vi "Stream Data.vi"(8 "error in (no error)":errorcluster, 10 "Data Type":string, 11 "Communication in":refnum<class "Communication.lvclass">) -> (0 "error out":errorcluster, 3 "Communication out":refnum<class "Communication.lvclass">)   [LabVIEW 2021, in "Communication.lvclass"]
uses:
  Communication.lvclass
  Data/Data.lvclass
  Controls/User Event Operation.ctl
  Downloads/Sample PC Template/Sample PC Template/Typedefs/Data.ctl
  Downloads/Sample PC Template/Sample PC Template/Sample PC Template.lvlib
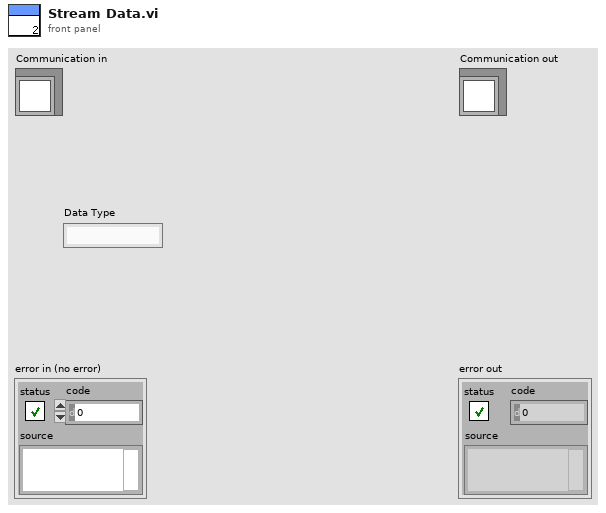
[diagram p1: front panel]
types:
  T1 = typedef "Sample PC Template.lvlib/Data.ctl" = cluster{"State":string, "Data":variant}
  T2 = typedef "User Event Operation.ctl" = enum16{"Obtain", "Generate", "Release"}
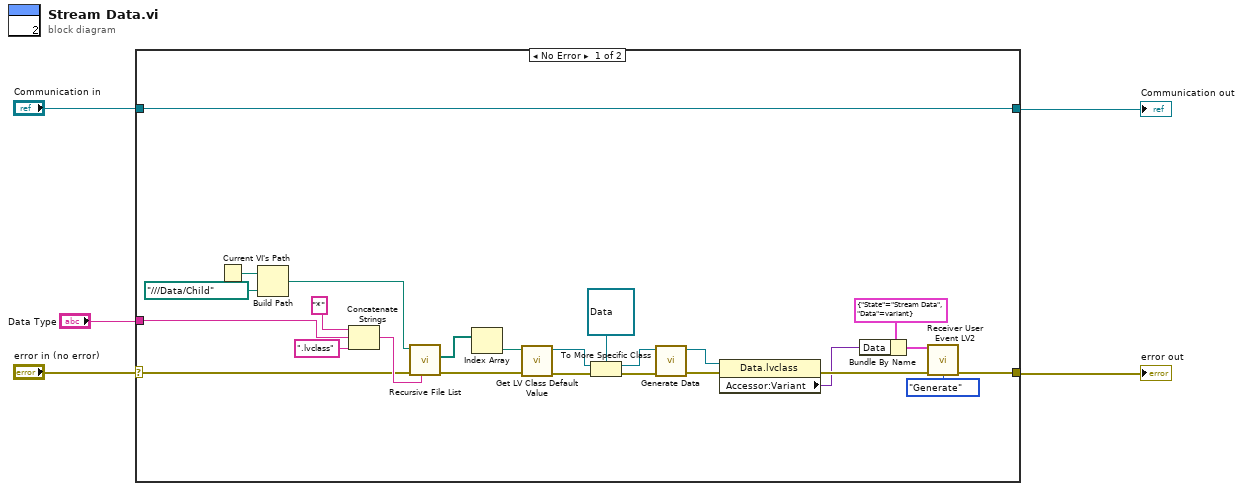
[diagram p0: block diagram]
diagram:
  n1 = case shown="No Error" "error in (no error)" {
    selector: "error in (no error)" -> [w8 w32]
    tunnel: [w7 w32] -> w4
    tunnel: [w30 w31] -> w2
    tunnel: "Communication in" -> [w30 w31]
    tunnel: "Data Type" -> [w6 _]
    frame No Error {
      n2 = Current VI's Path() -> (path=w29:path)
      n3 = Build Path(base path=w29, name or relative path=path "../../../Data/Child") -> (appended path=w13:path)
      n4 = Concatenate Strings("*" ("string"), w6, ".lvclass" ("string")) -> (w10:string)
      n5 = call <vilib>:"Recursive File List.vi"("pattern"=w10, "error in (no error)"=w8, "Folder Path"=w13) -> ("error out"=w28:errorcluster, "All Files in Dir"=w27:path[])  [unwired: 4 in, 3 out]
      n6 = Index Array(array=w27) -> (element=w9:path)  [unwired: 1 in]
      n7 = call <vilib>:"Get LV Class Default Value.vi"("error in (no error)"=w28, "class path"=w9) -> ("error out"=w25:errorcluster, "object"=w23:refnum<class>)  [unwired: 8 in]
      n8 = To More Specific Class(target class=refnum<class "Data.lvclass"> refnum ("Data.lvclass"), reference=w23, error in=w25) -> (specific class reference=w21:refnum<class "Data.lvclass">, error out=w22:errorcluster)
      n9 = call-dynamic "Generate Data.vi"("error in (no error)"=w22, "Data in"=w21) -> ("error out"=w20:errorcluster, "Data out"=w19:refnum<class "Data.lvclass">)  [unwired: 8 in]
      n10 = property class="Data.lvclass"(reference=w19, error in=w20) -> (error out=w18:errorcluster, "Accessor:Variant"=w15:variant)  [unwired: 1 out]
      n11 = Bundle By Name(cluster=T1 {"State"="Stream Data", "Data"=variant} ("Data"), "Data"=w15) -> (w14:T1)
      n12 = call "Receiver User Event LV2.vi"("Data"=w14, "Error In"=w18, "Operation"=User_Event_Operation."Generate") -> ("Error Out"=w7:errorcluster)  [unwired: 11 in, 1 out]
    }
    frame Error {
    }
  }
  "error out" <- w4
  "Communication out" <- w2
